vi "WILT Filename Generate SS.vi"(10 "name or relative path":string, 11 "path":path) -> (2 "file or folder exists?":bool, 3 "appended path":path)   [LabVIEW 2016]
panel:
  out "error out":errorcluster
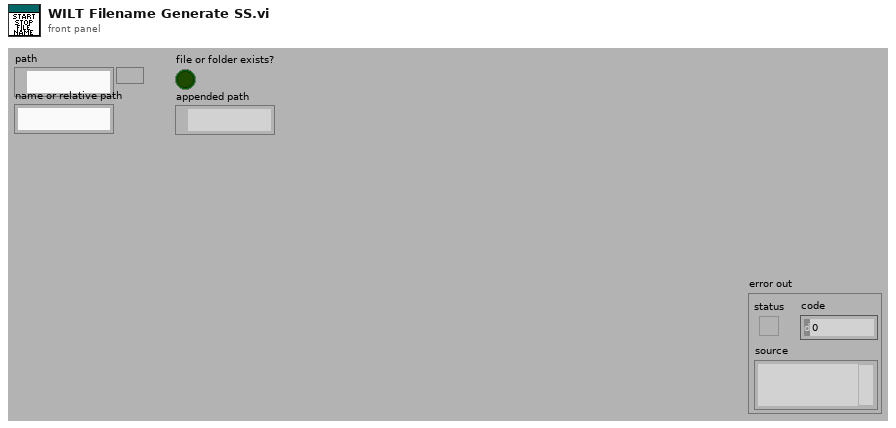
[diagram p1: front panel]
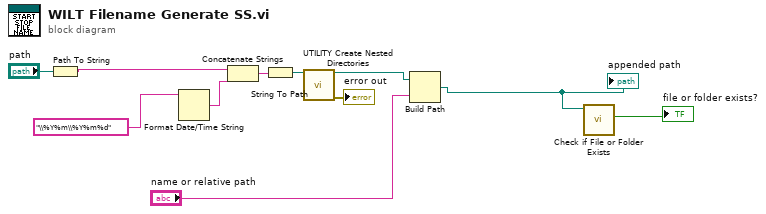
[diagram p0: block diagram]
diagram:
  n1 = Path To String(path="path") -> (string=w4:string)
  n2 = Format Date/Time String(time format string (%c)="\\%Y%m\\%Y%m%d") -> (date/time string=w6:string)  [unwired: 2 out]
  n3 = Concatenate Strings(w4, w6) -> (w5:string)
  n4 = String To Path(string=w5) -> (path=w7:path)
  n5 = call "UTILITY Create Nested Directories.vi"("path to create"=w7) -> ("created path"=w8:path, "error out"=→"error out":errorcluster)  [unwired: 12 in, 1 out]
  n6 = Build Path(base path=w8, name or relative path="name or relative path") -> (appended path=w9:path)
  "appended path" <- w9
  n7 = call <vilib>:"Check if File or Folder Exists.vi"("path"=w9) -> ("file or folder exists?"=→"file or folder exists?":bool)  [unwired: 8 in, 2 out]
